vi "系列号查询.vi"() -> ()   [LabVIEW 2016, in "斯坦道多参数.lvlib"]
panel:
  in  "传感器系列号":T1
  in  "布尔":bool
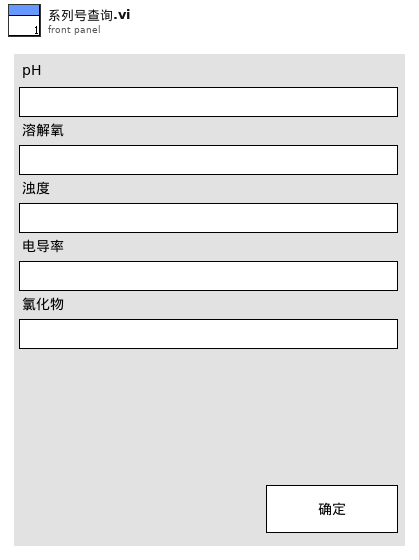
[diagram p1: front panel]
types:
  T1 = cluster{"pH":string, "溶解氧":string, "浊度":string, "电导率":string, "ORP":string, "叶绿素a":string, "藻密度":string, "氯化物":string}
  T2 = typedef "斯坦道多参数.lvlib/探头类型.ctl" = enum16{"禹山", "国弘", "纳清", "STD"}
  T3 = cluster{"pH探头选择":T2, "DO探头选择":T2, "电导率探头选择":T2, "浊度探头选择":T2, "悬浮物探头选择":T2, "叶绿素a探头选择":T2, "蓝绿藻探头选择":T2, "orp探头选择":T2, "COD探头选择":T2, "DO2探头选择":T2, "氨氮探头选择":T2, "水中油探头选择":T2, "余氯探头选择":T2}
  T4 = enum16{"null", "pH", "DO", "浊度", "电导率", "叶绿素a", "DO2"}
  T5 = cluster{"电极状态标志":u16, "电极型号标志":u16, "酸碱度测量值":sgl, "温度测量值":sgl, "酸碱度信号值":sgl, "温度信号值":sgl, "酸碱度偏移修正值":sgl, "温度偏移修正值":sgl, "手动温度补偿值":sgl, "酸碱度电极零点":sgl, "酸碱度电极斜率":sgl, "第1点标准值记录":sgl, "第1点信号值记录":sgl, "第1点温度值记录":sgl, "第2点标准值记录":sgl, "第2点信号值记录":sgl, "第2点温度值记录":sgl, "命令滤波设定":u16, "温度模式":enum16{"ATC", "MTC"}, "生产批次":u16, "电极序号":u16, "串口地址":u16, "串口波特率":enum16{"9600", "19200", "115200"}, "串口校验位":enum16{"NONE", "ODD", "EVEN"}, "串口停止位":enum16{"1bit", "2bit"}, "第一点标准值":sgl, "第二点标准值":sgl}
  T6 = cluster{"报警码":u16, "pH数值":sgl, "0X0003_NC":sgl, "温度数据":sgl, "pH原始信号 mv":sgl, "0X0009_NC":string, "产品名称":string, "序列号":string, "硬件版本":string, "软件版本":string, "通讯地址":u16, "波特率":u16, "设备类型":u16, "0X0026_NC":string, "第一点原始数据":sgl, "第一点校准数据":sgl, "第二点原始数据":sgl, "第二点校准数据":sgl, "探头校准命令":u16, "温度校准参数":sgl, "温度校准命令":u16}
  T7 = cluster{"电极状态标志":u16, "电极型号标志":u16, "溶解氧测量值":sgl, "温度测量值":sgl, "溶解氧饱和度值":sgl, "盐度补偿值":sgl, "大气压补偿值":sgl, "溶解氧偏移修正值":sgl, "温度偏移修正值":sgl, "手动温度补偿值":sgl, "溶解氧电极零点":sgl, "溶解氧电极斜率":sgl, "第1点标准值记录":sgl, "第1点信号值记录":sgl, "第1点温度值记录":sgl, "第2点标准值记录":sgl, "第2点信号值记录":sgl, "第2点温度值记录":sgl, "命令滤波设定":u16, "温度模式":enum16{"ATC", "MTC"}, "生产批次":u16, "电极序号":u16, "串口地址":u16, "串口波特率":enum16{"9600", "19200", "115200"}, "串口校验位":enum16{"NONE", "ODD", "EVEN"}, "串口停止位":enum16{"1bit", "2bit"}, "第一点标准值":sgl, "第二点标准值":sgl}
  T8 = cluster{"报警码":u16, "溶解氧数值（mg/L）":sgl, "溶解氧数据（%）":sgl, "温度数据":sgl, "溶解氧原始信号 nA":sgl, "大气压力":sgl, "盐度":sgl, "0X0009_NC":string, "产品名称":string, "序列号":string, "硬件版本":string, "软件版本":string, "通讯地址":u16, "波特率":u16, "设备类型":u16, "0X0026_NC":string, "第一点原始数据":sgl, "第一点校准数据":sgl, "第二点原始数据":sgl, "第二点校准数据":sgl, "探头校准命令":u16, "温度校准参数":sgl, "温度校准命令":u16}
  T9 = cluster{"电极状态标志":u16, "电极型号标志":u16, "浊度测量值":sgl, "温度测量值":sgl, "浊度信号值":sgl, "浊度偏移修正值":sgl, "温度偏移修正值":sgl, "手动温度补偿值":sgl, "浊度电极零点":sgl, "浊度电极斜率":sgl, "清洁周期":u16, "命令滤波设定":u16, "温度模式":enum16{"ATC", "MTC"}, "生产批次":u16, "电极序号":u16, "串口地址":u16, "串口波特率":enum16{"9600", "19200", "115200"}, "串口校验位":enum16{"NONE", "ODD", "EVEN"}, "串口停止位":enum16{"1bit", "2bit"}, "第一点标准值":sgl, "第二点标准值":sgl, "第三点标准值":sgl}
  T10 = cluster{"报警码":u16, "浊度数值 NTU":sgl, "温度数据":sgl, "原始光强数值":u16, "量程":u16, "平均次数":u16, "清扫模式":u16, "清扫次数":u16, "清扫间隔分钟":u16, "0X000B_NC":string, "产品名称":string, "序列号":string, "硬件版本":string, "软件版本":string, "通讯地址":u16, "波特率":u16, "设备类型":u16, "0X0026_NC":string, "校准量程":u16, "第一点原始光强":u16, "第一点校准数据":sgl, "第二点原始光强":u16, "第二点校准数据":sgl, "第三点原始光强":u16, "第三点校准数据":sgl, "探头校准命令":u16, "温度校准参数":sgl, "温度校准命令":u16}
  T11 = cluster{"电极状态标志":u16, "电极型号标志":u16, "电导率测量值":sgl, "温度测量值":sgl, "电导率信号值":sgl, "温度信号值":sgl, "温度补偿系数":sgl, "电导率偏移修正值":sgl, "温度偏移修正值":sgl, "手动温度补偿值":sgl, "电导率电极零点":sgl, "电导率电极斜率":sgl, "命令滤波设定":u16, "温度模式":enum16{"ATC", "MTC"}, "生产批次":u16, "电极序号":u16, "串口地址":u16, "串口波特率":enum16{"9600", "19200", "115200"}, "串口校验位":enum16{"NONE", "ODD", "EVEN"}, "串口停止位":enum16{"1bit", "2bit"}, "第一点标准值":sgl, "第二点标准值":sgl}
  T12 = cluster{"报警码":u16, "电导率数据（uS/cm）":sgl, "0x0003 NC":sgl, "温度数据":sgl, "电导率原始信号电阻":sgl, "当前量程":u16, "温度补偿系数":sgl, "0X0009_NC":string, "产品名称":string, "序列号":string, "硬件版本":string, "软件版本":string, "通讯地址":u16, "波特率":u16, "设备类型":u16, "0X0026_NC":string, "第一点原始数据":sgl, "第一点校准数据":sgl, "0X0035_NC":sgl, "0X0037_NC":sgl, "探头校准命令":u16, "温度校准参数":sgl, "温度校准命令":u16}
  T13 = cluster{"电极状态标志":u16, "电极型号标志":u16, "测量值":sgl, "温度测量值":sgl, "信号值":sgl, "温度信号值":sgl, "000AH_NC":sgl, "偏移修正值":sgl, "温度偏移修正值":sgl, "手动温度补偿值":sgl, "命令滤波设定":u16, "温度模式":enum16{"ATC", "MTC"}, "生产批次":u16, "传感器序号":u16, "串口地址":u16, "串口波特率":enum16{"9600", "19200", "115200"}, "串口校验位":enum16{"NONE", "ODD", "EVEN"}, "串口停止位":enum16{"1bit", "2bit"}}
  T14 = cluster{"报警码":u16, "叶绿素a":sgl, "温度数据":sgl, "原始光强数值":u16, "量程":u16, "平均次数":u16, "清扫模式":u16, "清扫次数":u16, "清扫间隔分钟":u16, "0X000B_NC":string, "产品名称":string, "序列号":string, "硬件版本":string, "软件版本":string, "通讯地址":u16, "波特率":u16, "设备类型":u16, "0X0026_NC":string, "校准量程":u16, "第一点原始光强":u16, "第一点校准数据":sgl, "第二点原始光强":u16, "第二点校准数据":sgl, "第三点原始光强":u16, "第三点校准数据":sgl, "探头校准命令":u16, "温度校准参数":sgl, "温度校准命令":u16}
  T15 = enum16{"null", "pH", "DO", "浊度", "电导率", "叶绿素a", "DO2", "藻密度"}
  T16 = cluster{"报警码":u16, "蓝绿藻":sgl, "温度数据":sgl, "原始光强数值":u16, "量程":u16, "平均次数":u16, "清扫模式":u16, "清扫次数":u16, "清扫间隔分钟":u16, "0X000B_NC":string, "产品名称":string, "序列号":string, "硬件版本":string, "软件版本":string, "通讯地址":u16, "波特率":u16, "设备类型":u16, "0X0026_NC":string, "校准量程":u16, "第一点原始光强":u16, "第一点校准数据":sgl, "第二点原始光强":u16, "第二点校准数据":sgl, "第三点原始光强":u16, "第三点校准数据":sgl, "探头校准命令":u16, "温度校准参数":sgl, "温度校准命令":u16}
  T17 = cluster{"电极状态标志":u16, "电极型号标志":u16, "测量值":sgl, "温度测量值":sgl, "信号值":sgl, "温度信号值":sgl, "偏移修正值":sgl, "温度偏移修正值":sgl, "手动温度补偿值":sgl, "电极零点":sgl, "电极斜率":sgl, "第1点标准值记录":sgl, "第1点信号值记录":sgl, "第1点温度值记录":sgl, "第2点标准值记录":sgl, "第2点信号值记录":sgl, "第2点温度值记录":sgl, "命令滤波设定":u16, "温度模式":enum16{"ATC", "MTC"}, "生产批次":u16, "电极序号":u16, "串口地址":u16, "串口波特率":enum16{"9600", "19200", "115200"}, "串口校验位":enum16{"NONE", "ODD", "EVEN"}, "串口停止位":enum16{"1bit", "2bit"}, "第一点标准值":sgl, "第二点标准值":sgl}
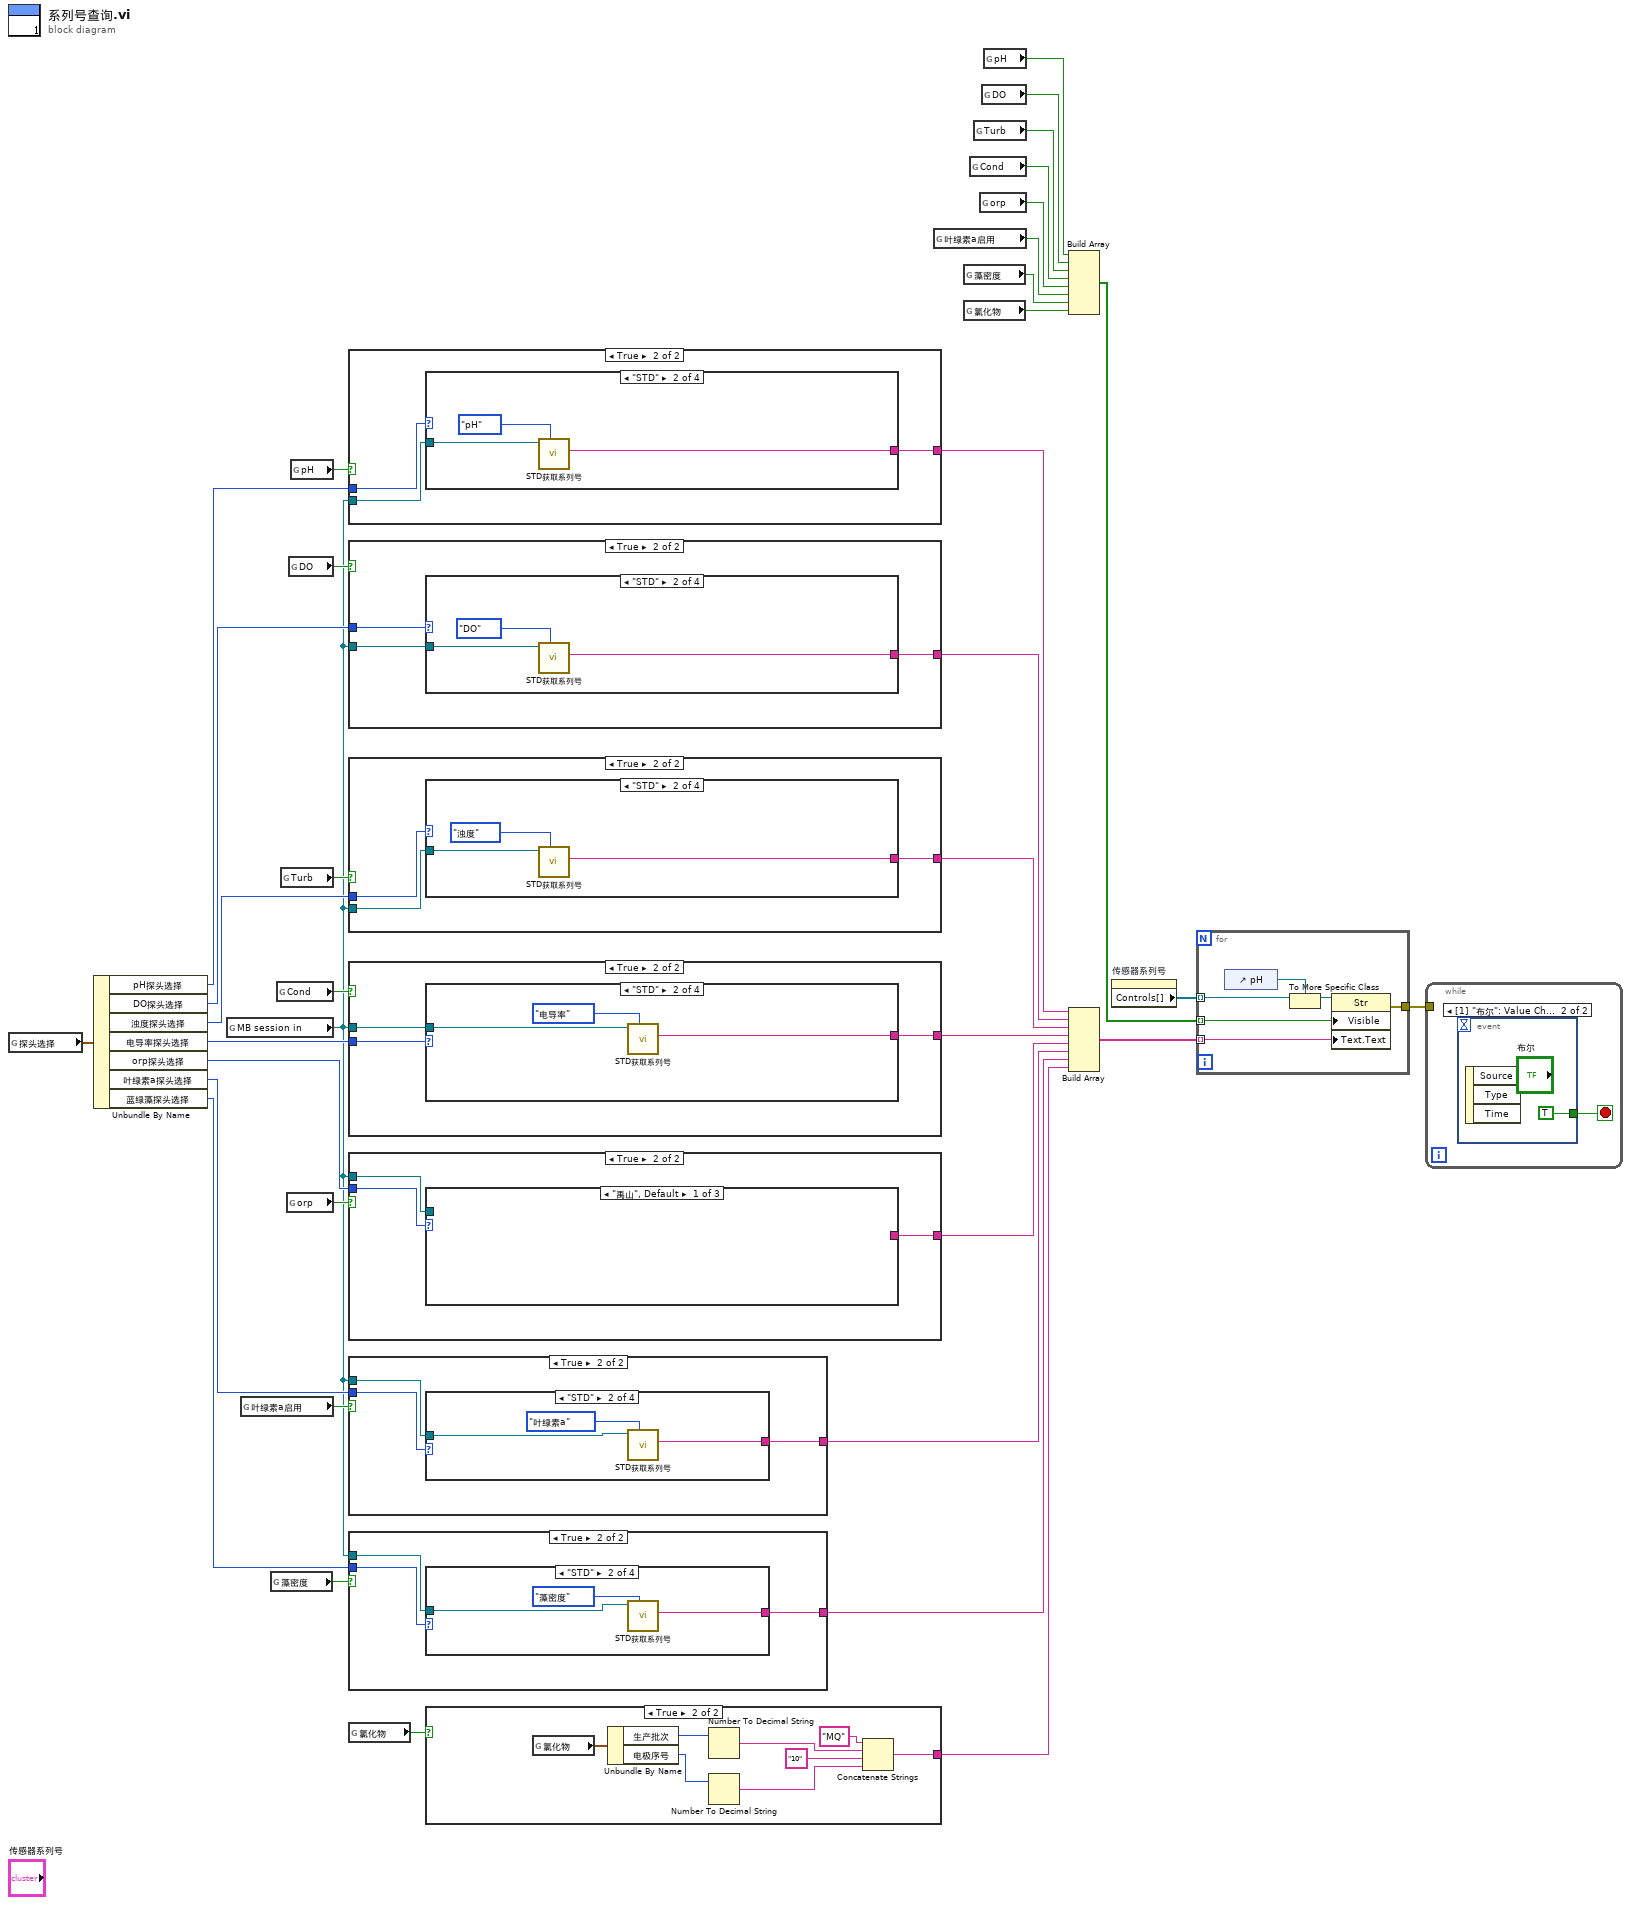
[diagram p0: block diagram]
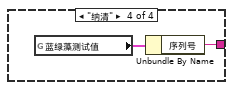
[diagram p6: hidden frame]
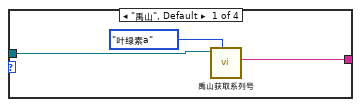
[diagram p8: hidden frame]
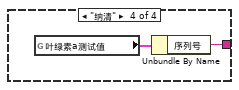
[diagram p10: hidden frame]
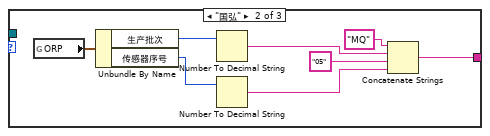
[diagram p12: hidden frame]
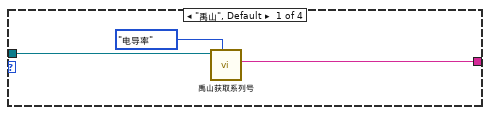
[diagram p15: hidden frame]
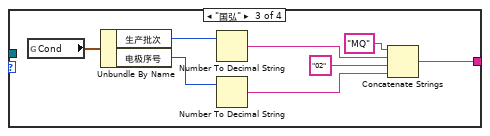
[diagram p16: hidden frame]
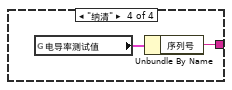
[diagram p17: hidden frame]
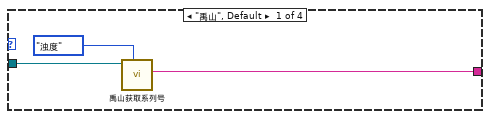
[diagram p19: hidden frame]
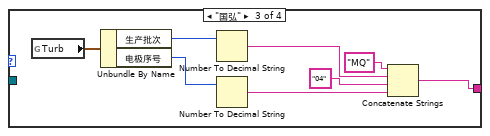
[diagram p20: hidden frame]
diagram:
  n1 = global read "断电保存变量.vi" "探头选择"() -> (w27:T3)
  n2 = Unbundle By Name(w27) -> ("pH探头选择"=w26:T2, "DO探头选择"=w24:T2, "浊度探头选择"=w22:T2, "电导率探头选择"=w19:T2, "orp探头选择"=w18:T2, "叶绿素a探头选择"=w16:T2, "蓝绿藻探头选择"=w12:T2)
  n3 = global read "多参数全局变量.vi" "MB session in"() -> (w13:refnum<class "MB_Master.lvclass">)
  n4 = global read "断电保存变量.vi" "叶绿素a启用"() -> (w15:bool)
  n5 = global read "断电保存变量.vi" "藻密度"() -> (w14:bool)
  n6 = global read "断电保存变量.vi" "Cond"() -> (w20:bool)
  n7 = global read "断电保存变量.vi" "Turb"() -> (w21:bool)
  n8 = global read "断电保存变量.vi" "orp"() -> (w17:bool)
  n9 = global read "断电保存变量.vi" "DO"() -> (w23:bool)
  n10 = global read "断电保存变量.vi" "pH"() -> (w25:bool)
  n11 = case shown="True" w25 {
    tunnel: w26 -> [_ w40]
    tunnel: [_ w39] -> w11
    tunnel: w13 -> [_ w38]
    frame False {
    }
    frame True {
      n12 = case shown="\"STD\"" w40 {
        tunnel: w38 -> [w43 w46 _ _]
        tunnel: [w42 w45 w50 w55] -> w39
        frame "禹山", Default {
          n13 = call "禹山获取系列号.vi"("探头"=T4."pH", "MB session in"=w43) -> ("SN"=w42:string)  [unwired: 7 in, 2 out]
        }
        frame "STD" {
          n14 = call "STD获取系列号.vi"("探头"=T4."pH", "MB session in"=w46) -> ("SN"=w45:string)  [unwired: 7 in, 2 out]
        }
        frame "国弘" {
          n15 = global read "国弘过程全局变量.vi" "pH"() -> (w51:T5)
          n16 = Unbundle By Name(w51) -> ("生产批次"=w52:u16, "电极序号"=w53:u16)
          n17 = Number To Decimal String(number=w52) -> (decimal integer string=w54:string)  [unwired: 1 in]
          n18 = Number To Decimal String(number=w53) -> (decimal integer string=w48:string)  [unwired: 1 in]
          n19 = Concatenate Strings("MQ" ("字符串"), w54, "01" ("字符串"), w48) -> (w50:string)
        }
        frame "纳清" {
          n20 = global read "纳清过程全局变量.vi" "pH测试值"() -> (w56:T6)
          n21 = Unbundle By Name(w56) -> ("序列号"=w55:string)
        }
      }
    }
  }
  n22 = case shown="True" w23 {
    tunnel: w24 -> [_ w59]
    tunnel: [_ w58] -> w10
    tunnel: w13 -> [_ w57]
    frame False {
    }
    frame True {
      n23 = case shown="\"STD\"" w59 {
        tunnel: w57 -> [w62 w65 _ _]
        tunnel: [w61 w63 w69 w74] -> w58
        frame "禹山", Default {
          n24 = call "禹山获取系列号.vi"("探头"=T4."DO", "MB session in"=w62) -> ("SN"=w61:string)  [unwired: 7 in, 2 out]
        }
        frame "STD" {
          n25 = call "STD获取系列号.vi"("探头"=T4."DO", "MB session in"=w65) -> ("SN"=w63:string)  [unwired: 7 in, 2 out]
        }
        frame "国弘" {
          n26 = global read "国弘过程全局变量.vi" "DO"() -> (w70:T7)
          n27 = Unbundle By Name(w70) -> ("生产批次"=w71:u16, "电极序号"=w72:u16)
          n28 = Number To Decimal String(number=w71) -> (decimal integer string=w73:string)  [unwired: 1 in]
          n29 = Number To Decimal String(number=w72) -> (decimal integer string=w67:string)  [unwired: 1 in]
          n30 = Concatenate Strings("MQ" ("字符串"), w73, "03" ("字符串"), w67) -> (w69:string)
        }
        frame "纳清" {
          n31 = global read "纳清过程全局变量.vi" "DO测试值"() -> (w75:T8)
          n32 = Unbundle By Name(w75) -> ("序列号"=w74:string)
        }
      }
    }
  }
  n33 = case shown="True" w21 {
    tunnel: w22 -> [_ w78]
    tunnel: [_ w77] -> w9
    tunnel: w13 -> [_ w76]
    frame False {
    }
    frame True {
      n34 = case shown="\"STD\"" w78 {
        tunnel: w76 -> [w81 w84 _ _]
        tunnel: [w80 w83 w88 w93] -> w77
        frame "禹山", Default {
          n35 = call "禹山获取系列号.vi"("探头"=T4."浊度", "MB session in"=w81) -> ("SN"=w80:string)  [unwired: 7 in, 2 out]
        }
        frame "STD" {
          n36 = call "STD获取系列号.vi"("探头"=T4."浊度", "MB session in"=w84) -> ("SN"=w83:string)  [unwired: 7 in, 2 out]
        }
        frame "国弘" {
          n37 = global read "国弘过程全局变量.vi" "Turb"() -> (w89:T9)
          n38 = Unbundle By Name(w89) -> ("生产批次"=w90:u16, "电极序号"=w91:u16)
          n39 = Number To Decimal String(number=w90) -> (decimal integer string=w92:string)  [unwired: 1 in]
          n40 = Number To Decimal String(number=w91) -> (decimal integer string=w86:string)  [unwired: 1 in]
          n41 = Concatenate Strings("MQ" ("字符串"), w92, "04" ("字符串"), w86) -> (w88:string)
        }
        frame "纳清" {
          n42 = global read "纳清过程全局变量.vi" "浊度测试值"() -> (w94:T10)
          n43 = Unbundle By Name(w94) -> ("序列号"=w93:string)
        }
      }
    }
  }
  n44 = case shown="True" w20 {
    tunnel: w19 -> [_ w97]
    tunnel: [_ w96] -> w8
    tunnel: w13 -> [_ w95]
    frame False {
    }
    frame True {
      n45 = case shown="\"STD\"" w97 {
        tunnel: w95 -> [w100 w103 _ _]
        tunnel: [w99 w102 w107 w112] -> w96
        frame "禹山", Default {
          n46 = call "禹山获取系列号.vi"("探头"=T4."电导率", "MB session in"=w100) -> ("SN"=w99:string)  [unwired: 7 in, 2 out]
        }
        frame "STD" {
          n47 = call "STD获取系列号.vi"("探头"=T4."电导率", "MB session in"=w103) -> ("SN"=w102:string)  [unwired: 7 in, 2 out]
        }
        frame "国弘" {
          n48 = global read "国弘过程全局变量.vi" "Cond"() -> (w108:T11)
          n49 = Unbundle By Name(w108) -> ("生产批次"=w109:u16, "电极序号"=w110:u16)
          n50 = Number To Decimal String(number=w109) -> (decimal integer string=w111:string)  [unwired: 1 in]
          n51 = Number To Decimal String(number=w110) -> (decimal integer string=w105:string)  [unwired: 1 in]
          n52 = Concatenate Strings("MQ" ("字符串"), w111, "02" ("字符串"), w105) -> (w107:string)
        }
        frame "纳清" {
          n53 = global read "纳清过程全局变量.vi" "电导率测试值"() -> (w113:T12)
          n54 = Unbundle By Name(w113) -> ("序列号"=w112:string)
        }
      }
    }
  }
  n55 = case shown="True" w17 {
    tunnel: w18 -> [_ w116]
    tunnel: [_ w115] -> w7
    tunnel: w13 -> [_ w114]
    frame False {
    }
    frame True {
      n56 = case shown="\"禹山\", Default" w116 {
        tunnel: w114 -> [_ _ _]
        tunnel: [_ w120 _] -> w115
        frame "禹山", Default {
        }
        frame "国弘" {
          n57 = global read "国弘过程全局变量.vi" "ORP"() -> (w121:T13)
          n58 = Unbundle By Name(w121) -> ("生产批次"=w122:u16, "传感器序号"=w123:u16)
          n59 = Number To Decimal String(number=w122) -> (decimal integer string=w124:string)  [unwired: 1 in]
          n60 = Number To Decimal String(number=w123) -> (decimal integer string=w118:string)  [unwired: 1 in]
          n61 = Concatenate Strings("MQ" ("字符串"), w124, "05" ("字符串"), w118) -> (w120:string)
        }
        frame "纳清" {
        }
      }
    }
  }
  n62 = case shown="True" w15 {
    tunnel: w16 -> [_ w127]
    tunnel: [_ w126] -> w6
    tunnel: w13 -> [_ w125]
    frame False {
    }
    frame True {
      n63 = case shown="\"STD\"" w127 {
        tunnel: w125 -> [w130 w133 _ _]
        tunnel: [w129 w132 _ w134] -> w126
        frame "禹山", Default {
          n64 = call "禹山获取系列号.vi"("探头"=T4."叶绿素a", "MB session in"=w130) -> ("SN"=w129:string)  [unwired: 7 in, 2 out]
        }
        frame "STD" {
          n65 = call "STD获取系列号.vi"("探头"=T4."叶绿素a", "MB session in"=w133) -> ("SN"=w132:string)  [unwired: 7 in, 2 out]
        }
        frame "国弘" {
        }
        frame "纳清" {
          n66 = global read "纳清过程全局变量.vi" "叶绿素a测试值"() -> (w135:T14)
          n67 = Unbundle By Name(w135) -> ("序列号"=w134:string)
        }
      }
    }
  }
  n68 = case shown="True" w14 {
    tunnel: w12 -> [_ w138]
    tunnel: [_ w137] -> w5
    tunnel: w13 -> [_ w136]
    frame False {
    }
    frame True {
      n69 = case shown="\"STD\"" w138 {
        tunnel: w136 -> [_ w141 _ _]
        tunnel: [_ w139 _ w142] -> w137
        frame "禹山", Default {
        }
        frame "STD" {
          n70 = call "STD获取系列号.vi"("探头"=T15."藻密度", "MB session in"=w141) -> ("SN"=w139:string)  [unwired: 7 in, 2 out]
        }
        frame "国弘" {
        }
        frame "纳清" {
          n71 = global read "纳清过程全局变量.vi" "蓝绿藻测试值"() -> (w143:T16)
          n72 = Unbundle By Name(w143) -> ("序列号"=w142:string)
        }
      }
    }
  }
  n73 = global read "断电保存变量.vi" "氯化物"() -> (w3:bool)
  n74 = case shown="True" w3 {
    tunnel: [_ w144] -> w2
    frame False {
    }
    frame True {
      n75 = global read "国弘过程全局变量.vi" "氯化物"() -> (w148:T17)
      n76 = Unbundle By Name(w148) -> ("生产批次"=w149:u16, "电极序号"=w150:u16)
      n77 = Number To Decimal String(number=w149) -> (decimal integer string=w151:string)  [unwired: 1 in]
      n78 = Number To Decimal String(number=w150) -> (decimal integer string=w146:string)  [unwired: 1 in]
      n79 = Concatenate Strings("MQ" ("字符串"), w151, "10" ("字符串"), w146) -> (w144:string)
    }
  }
  n80 = global read "断电保存变量.vi" "叶绿素a启用"() -> (w32:bool)
  n81 = global read "断电保存变量.vi" "藻密度"() -> (w31:bool)
  n82 = global read "断电保存变量.vi" "氯化物"() -> (w1:bool)
  n83 = global read "断电保存变量.vi" "Cond"() -> (w34:bool)
  n84 = global read "断电保存变量.vi" "Turb"() -> (w35:bool)
  n85 = global read "断电保存变量.vi" "orp"() -> (w33:bool)
  n86 = global read "断电保存变量.vi" "DO"() -> (w36:bool)
  n87 = global read "断电保存变量.vi" "pH"() -> (w37:bool)
  n88 = Build Array(w37, w36, w35, w34, w33, w32, w31, w1) -> (w29:bool[])
  n89 = Build Array(w11, w10, w9, w8, w7, w6, w5, w2) -> (w4:string[])
  n90 = property on="传感器系列号" class="Clust (strict)"() -> ("Controls[]"=w30:refnum<vi>[])  [unwired: 2 in, 2 out]
  n91 = for {
    tunnel: w30 -> [w155] mode=indexing
    tunnel: w29 -> [w157] mode=indexing
    tunnel: [w156] -> w28
    tunnel: w4 -> [w152] mode=indexing
    n92 = control-ref of="pH"() -> (w154:refnum<vi>)
    n93 = To More Specific Class(target class=w154, reference=w155) -> (specific class reference=w153:refnum<vi>)  [unwired: 1 in, 1 out]
    n94 = property class="Str"(reference=w153, "Visible"=w157, "Text.Text"=w152) -> (error out=w156:errorcluster)  [unwired: 1 in, 1 out]
  }
  n95 = while {
    tunnel: w28 -> [_]
    stop <- w158 stop-if-true
    n96 = event shown="[1] \"布尔\": Value Change;  Panel Close" {
      selector: _ -> [_ _]
      dyn-events: _ -> [_ _]
      timeout: _ -> [_ _]
      tunnel: [_ TRUE] -> w158
      event Timeout {
        n97 = event-data() -> ()  [unwired: 1 in, 3 out]
      }
      event "布尔": Value Change; Panel Close {
        n98 = event-data() -> ()  [unwired: 1 in, 3 out]
      }
    }
  }
